vi "pp2_log_trialTypes.vi"(10 "Trial Types File Path":path, 11 "Trial Types":T1[](array[typedef]) {"DAQ Amplitude (V)" min=0.0 max=5.0 format="%_6g"; "Shock (mA)" min=-1.0 max=5.0; "Trial Weight" step=1; "Duration (ms)" min=0.0 max=1.0; "Trial Type Number" min=1 max=256 step=1}) -> ()   [LabVIEW 2013]
uses:
  LV3/impl/pp3_CTL_Trial.ctl
  LV3/impl/pp3_CTL_TrialType.ctl
  labolabo2/waveforms/WFTypes.ctl
  <vilib>/Utility/file.llb/Write To Spreadsheet File (string).vi
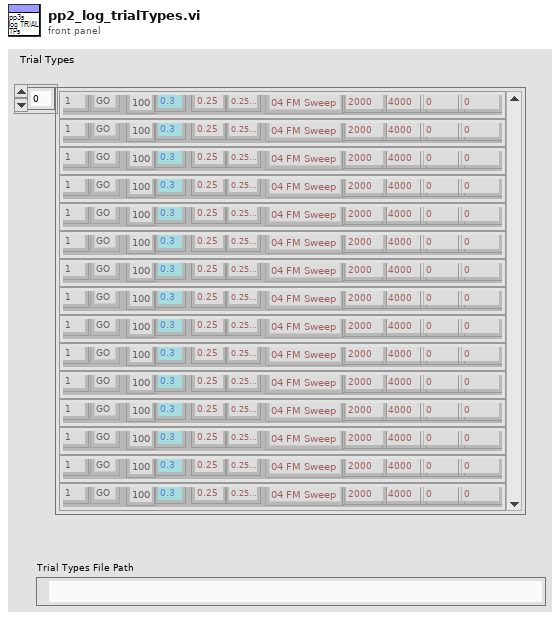
[diagram p1: front panel]
types:
  T1 = typedef "pp3_CTL_Trial.ctl" = cluster{"Trial Type Number":i16, "Trial Type":T2, "Trial Weight":u32, "Shock (mA)":dbl, "Duration (ms)":dbl, "Sound Type":T3, "Stim P1":dbl, "Stim P2":dbl, "Stim P3":dbl, "Stim P4":dbl, "DAQ Amplitude (V)":dbl}
  T2 = typedef "pp3_CTL_TrialType.ctl" = enum16{"OFF", "GO", "NOGO", "TEST"}
  T3 = typedef "WFTypes.ctl" = enum16{"00 NULL", "01 DC", "02 Noise", "03 Pure Tone", "04 FM Sweep"}
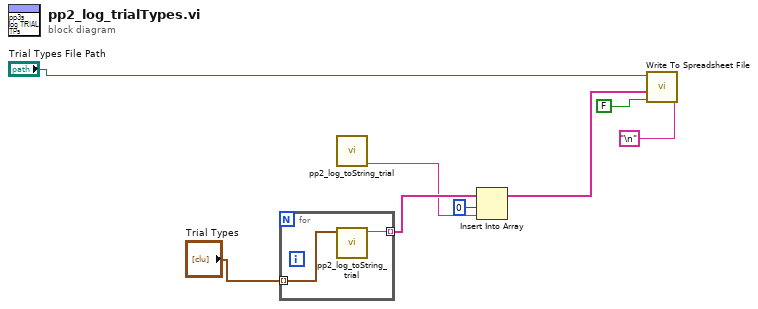
[diagram p0: block diagram]
diagram:
  n1 = for {
    tunnel: "Trial Types" -> [w10] mode=indexing
    tunnel: [w9] -> w5 mode=indexing
    n2 = call "pp2_log_toString_trial.vi"("Trial in"=w10) -> ("spreadsheet string"=w9:string)  [unwired: 9 in, 1 out]
  }
  n3 = call "pp2_log_toString_trial.vi"() -> ("TRIALMEMO String"=w4:string)  [unwired: 10 in, 1 out]
  n4 = Insert Into Array(array=w5, index=0, new element=w4) -> (w2:string[])
  n5 = call-poly <vilib>:"Write To Spreadsheet File.vi"("delimiter (\\t)"="\n" ("delimiter (\\t)"), "append to file? (new file:F)"=FALSE, "1D data"=w2, "file path (dialog if empty)"="Trial Types File Path") -> ()  [unwired: 4 in, 1 out]
